vi "XSP3_ControlAcquire.vi"(6 "Acquire":enum16{"Stop", "Start"}(ring) caption="ControlAcquire", 8 "ErrorIn":errorcluster, 11 "ProcessIn":string="XSPRESS3-EXAMPLE" caption="ProcessName") -> (0 "ErrorOut":errorcluster, 2 "Status":bool, 3 "ProcessOut":string caption="ProcessName")   [LabVIEW 2010]
uses:
  Program Files/National Instruments/LabVIEW 2017/user.lib/caLab/Private/Put_I16_PV.vi
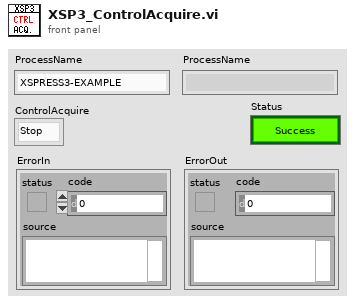
[diagram p1: front panel]
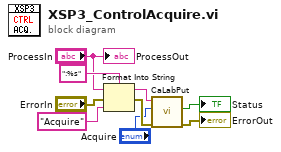
[diagram p0: block diagram]
diagram:
  n1 = Format Into String(format string=":%s" ("PV"), initial string="ProcessIn", error in="ErrorIn", "Acquire" ("PV")) -> (resulting string=w3:string, error out=w4:errorcluster)
  n2 = call-poly "CaLabPut.vi"("Error in (no error)"=w4, "Value"="Acquire", "PV Name"=w3) -> ("Error out"=→"ErrorOut":errorcluster, "Status"=→"Status":bool)  [unwired: 5 in, 2 out]
  "ProcessOut" <- "ProcessIn"
